vi "Variant to DBL.vi"(11 "Variant":variant) -> (2 "Value as DBL":dbl, 3 "Type":T1)   [LabVIEW 2022 SP3, in "Interlocks.lvlib"]
uses:
  Interlocks.lvlib
  Controls/Data Type.ctl
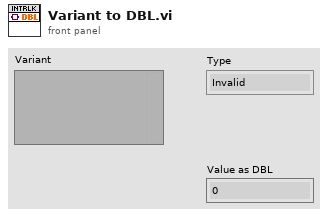
[diagram p1: front panel]
types:
  T1 = typedef "Interlocks.lvlib/Data Type.ctl" = enum8{"Invalid", "Boolean", "DBL", "I64", "U64"}
  T2 = enum8{"<Null>", "I8", "I16", "I32", "I64", "U8", "U16", "U32", "U64", "SGL", "DBL", "EXT", "CSG", "CDB", "CXT", "0x0F", "0x10", "0x11", "0x12", "0x13", "0x14", "Enum U8", "Enum U16", "Enum U32", "Enum U64", "SGL PQ", "DBL PQ", "EXT PQ", "CSG PQ", "CDB PQ", "CXT PQ", "0x1F", "0x20", "Boolean", "0x22", "0x23", "0x24", "0x25", "0x26", "0x27", "0x28", "0x29", "0x2A", "0x2B", "0x2C", "0x2D", "0x2E", "0x2F", "String", "0x31", "Path", "Pict", "0x34", "0x35", "0x36", "DAQ", "0x38", "0x39", "0x3A", "0x3B", "0x3C", "0x3D", "0x3E", "0x3F", "Array", "0x41", "0x42", "0x43", "0x44", "0x45", "0x46", "0x47", "0x48", "0x49", "0x4A", "0x4B", "0x4C", "0x4D", "0x4E", "0x4F", "Cluster", "0x51", "0x52", "Variant", "Waveform", "0x55", "0x56", "0x57", "0x58", "0x59", "0x5A", "0x5B", "0x5C", "0x5D", "0x5E", "Fixed Point", "0x60", "0x61", "0x62", "0x63", "0x64", "0x65", "0x66", "0x67", "0x68", "0x69", "0x6A", "0x6B", "0x6C", "0x6D", "0x6E", "0x6F", "Refnum", "0x71", "0x72", "Set Collection", "Map Collection"}
  T3 = cluster{"length":u16, "private":u8, "type":enum8{"<Null>", "I8", "I16", "I32", "I64", "U8", "U16", "U32", "U64", "SGL", "DBL", "EXT", "CSG", "CDB", "CXT", "0x0F", "0x10", "0x11", "0x12", "0x13", "0x14", "Enum U8", "Enum U16", "Enum U32", "Enum U64", "SGL PQ", "DBL PQ", "EXT PQ", "CSG PQ", "CDB PQ", "CXT PQ", "0x1F", "0x20", "Boolean", "0x22", "0x23", "0x24", "0x25", "0x26", "0x27", "0x28", "0x29", "0x2A", "0x2B", "0x2C", "0x2D", "0x2E", "0x2F", "String", "0x31", "Path", "Pict", "0x34", "0x35", "0x36", "DAQ", "0x38", "0x39", "0x3A", "0x3B", "0x3C", "0x3D", "0x3E", "0x3F", "Array", "0x41", "0x42", "0x43", "0x44", "0x45", "0x46", "0x47", "0x48", "0x49", "0x4A", "0x4B", "0x4C", "0x4D", "0x4E", "0x4F", "Cluster", "0x51", "0x52", "Variant", "Waveform", "0x55", "0x56", "0x57", "0x58", "0x59", "0x5A", "0x5B", "0x5C", "0x5D", "0x5E", "Fixed Point", "0x60", "0x61", "0x62", "0x63", "0x64", "0x65", "0x66", "0x67", "0x68", "0x69", "0x6A", "0x6B", "0x6C", "0x6D", "0x6E", "0x6F", "Refnum", "0x71", "0x72", "Set Collection", "Map Collection"}, "# elements":u16}
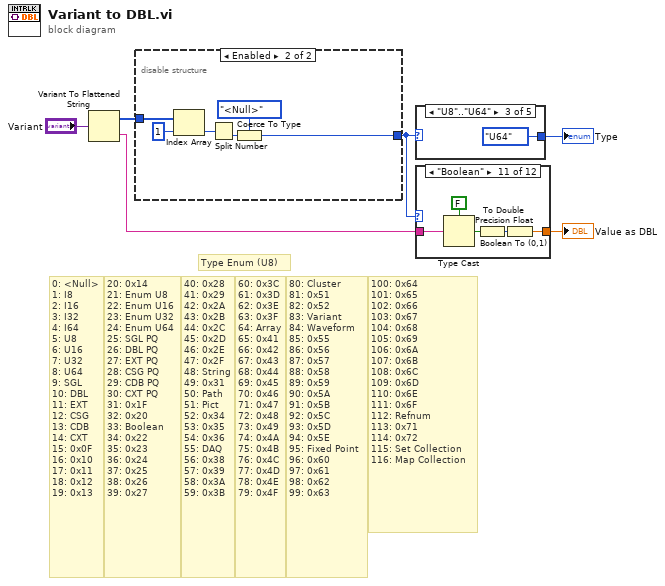
[diagram p0: block diagram]
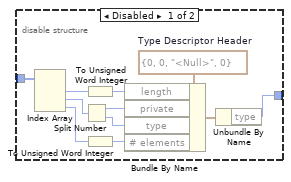
[diagram p2: hidden frame]
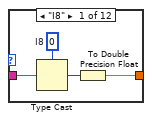
[diagram p3: hidden frame]
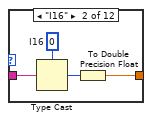
[diagram p4: hidden frame]
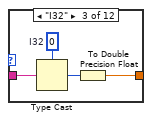
[diagram p5: hidden frame]
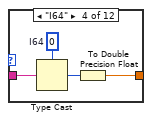
[diagram p6: hidden frame]
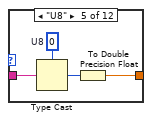
[diagram p7: hidden frame]
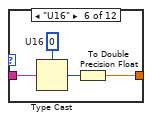
[diagram p8: hidden frame]
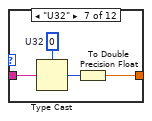
[diagram p9: hidden frame]
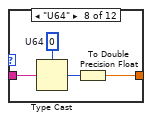
[diagram p10: hidden frame]
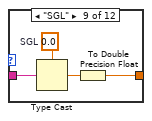
[diagram p11: hidden frame]
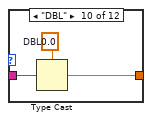
[diagram p12: hidden frame]
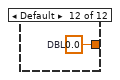
[diagram p13: hidden frame]
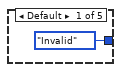
[diagram p14: hidden frame]
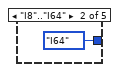
[diagram p15: hidden frame]
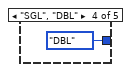
[diagram p16: hidden frame]
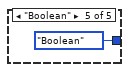
[diagram p17: hidden frame]
diagram:
  # "Type Enum (U8)"
  # "100: 0x64\n101: 0x65\n102: 0x66\n103: 0x67\n104: 0x68\n105: 0x69\n106: 0x6A\n107: 0x6B\n108: 0x6C\n109: 0x6D\n110: 0x6E\n111: 0x6F\n112: Refnum\n113: 0x71\n114: 0x72\n115: Set Collection\n116: Map Collection"
  # "80: Cluster\n81: 0x51\n82: 0x52\n83: Variant\n84: Waveform\n85: 0x55\n86: 0x56\n87: 0x57\n88: 0x58\n89: 0x59\n90: 0x5A\n91: 0x5B\n92: 0x5C\n93: 0x5D\n94: 0x5E\n95: Fixed Point\n96: 0x60\n97: 0x61\n98: 0x62\n99: 0x63"
  # "60: 0x3C\n61: 0x3D\n62: 0x3E\n63: 0x3F\n64: Array\n65: 0x41\n66: 0x42\n67: 0x43\n68: 0x44\n69: 0x45\n70: 0x46\n71: 0x47\n72: 0x48\n73: 0x49\n74: 0x4A\n75: 0x4B\n76: 0x4C\n77: 0x4D\n78: 0x4E\n79: 0x4F"
  # "40: 0x28\n41: 0x29\n42: 0x2A\n43: 0x2B\n44: 0x2C\n45: 0x2D\n46: 0x2E\n47: 0x2F\n48: String\n49: 0x31\n50: Path\n51: Pict\n52: 0x34\n53: 0x35\n54: 0x36\n55: DAQ\n56: 0x38\n57: 0x39\n58: 0x3A\n59: 0x3B"
  # "20: 0x14\n21: Enum U8\n22: Enum U16\n23: Enum U32\n24: Enum U64\n25: SGL PQ\n26: DBL PQ\n27: EXT PQ\n28: CSG PQ\n29: CDB PQ\n30: CXT PQ\n31: 0x1F\n32: 0x20\n33: Boolean\n34: 0x22\n35: 0x23\n36: 0x24\n37: 0x25\n38: 0x26 \n39: 0x27"
  # "0: <Null>\n1: I8\n2: I16\n3: I32\n4: I64\n5: U8\n6: U16\n7: U32\n8: U64\n9: SGL\n10: DBL\n11: EXT\n12: CSG\n13: CDB\n14: CXT\n15: 0x0F\n16: 0x10\n17: 0x11\n18: 0x12\n19: 0x13"
  n1 = Variant To Flattened String(Variant="Variant") -> (data string=w2:string, 1:w5:i16[])
  n2 = disable-structure shown="Enabled" {
    disable-tunnel: w5 -> [w9 w23]
    disable-tunnel: [w7 w18] -> w3
    frame Disabled {
      w12 = T3 {"length"=0, "private"=0, "type"=enum."<Null>", "# elements"=0}  # Type Descriptor Header
      n3 = Index Array(array=w9) -> (element #1=w13:i16, element #2=w16:i16, element #3=w17:i16)  [unwired: 3 in]
      n4 = Split Number(x=w16) -> (hi(x)=w14:u8, lo(x)=w15:u8)
      n5 = To Unsigned Word Integer(number=w13) -> (unsigned 16bit integer=w10:u16)
      n6 = To Unsigned Word Integer(number=w17) -> (unsigned 16bit integer=w11:u16)
      n7 = Bundle By Name(cluster=w12, "length"=w10, "private"=w14, "type"=w15, "# elements"=w11) -> (w8:T3)
      n8 = Unbundle By Name(w8) -> ("type"=w7:T2)
    }
    frame Enabled {
      n9 = Index Array(array=w23, index=1) -> (element=w21:i16)
      n10 = Split Number(x=w21) -> (lo(x)=w20:u8)  [unwired: 1 out]
      n11 = Coerce To Type(0:w20, 1:T2."<Null>" ("type")) -> (2:w18:T2)
    }
  }
  n12 = case shown="\"U8\"..\"U64\"" w3 {
    tunnel: [Data_Type."Invalid" ("Type") Data_Type."I64" ("Type") Data_Type."U64" ("Type") Data_Type."DBL" ("Type") Data_Type."Boolean" ("Type")] -> w4
    frame Default {
    }
    frame "I8".."I64" {
    }
    frame "U8".."U64" {
    }
    frame "SGL", "DBL" {
    }
    frame "Boolean" {
    }
  }
  "Type" <- w4
  n13 = case shown="\"Boolean\"" w3 {
    tunnel: w2 -> [w32 w36 w40 w43 w48 w52 w56 w60 w64 w66 w72 _]
    tunnel: [w29 w33 w37 w41 w45 w49 w53 w57 w61 w65 w68 w73] -> w1
    frame "I8" {
      w31 = i8 0  # I8
      n14 = Type Cast(type=w31, x=w32) -> (*(type *) &x=w30:i8)
      n15 = To Double Precision Float(number=w30) -> (double precision float=w29:dbl)
    }
    frame "I16" {
      w35 = i16 0  # I16
      n16 = Type Cast(type=w35, x=w36) -> (*(type *) &x=w34:i16)
      n17 = To Double Precision Float(number=w34) -> (double precision float=w33:dbl)
    }
    frame "I32" {
      w39 = 0  # I32
      n18 = Type Cast(type=w39, x=w40) -> (*(type *) &x=w38:i32)
      n19 = To Double Precision Float(number=w38) -> (double precision float=w37:dbl)
    }
    frame "I64" {
      w44 = i64 0  # I64
      n20 = Type Cast(type=w44, x=w43) -> (*(type *) &x=w42:i64)
      n21 = To Double Precision Float(number=w42) -> (double precision float=w41:dbl)
    }
    frame "U8" {
      w47 = u8 0  # U8
      n22 = Type Cast(type=w47, x=w48) -> (*(type *) &x=w46:u8)
      n23 = To Double Precision Float(number=w46) -> (double precision float=w45:dbl)
    }
    frame "U16" {
      w51 = u16 0  # U16
      n24 = Type Cast(type=w51, x=w52) -> (*(type *) &x=w50:u16)
      n25 = To Double Precision Float(number=w50) -> (double precision float=w49:dbl)
    }
    frame "U32" {
      w55 = u32 0  # U32
      n26 = Type Cast(type=w55, x=w56) -> (*(type *) &x=w54:u32)
      n27 = To Double Precision Float(number=w54) -> (double precision float=w53:dbl)
    }
    frame "U64" {
      w59 = u64 0  # U64
      n28 = Type Cast(type=w59, x=w60) -> (*(type *) &x=w58:u64)
      n29 = To Double Precision Float(number=w58) -> (double precision float=w57:dbl)
    }
    frame "SGL" {
      w63 = sgl 0.0  # SGL
      n30 = Type Cast(type=w63, x=w64) -> (*(type *) &x=w62:sgl)
      n31 = To Double Precision Float(number=w62) -> (double precision float=w61:dbl)
    }
    frame "DBL" {
      w67 = 0.0  # DBL
      n32 = Type Cast(type=w67, x=w66) -> (*(type *) &x=w65:dbl)
    }
    frame "Boolean" {
      n33 = Type Cast(type=FALSE, x=w72) -> (*(type *) &x=w70:bool)
      n34 = Boolean To (0,1)(Boolean=w70) -> (0, 1=w69:i16)
      n35 = To Double Precision Float(number=w69) -> (double precision float=w68:dbl)
    }
    frame Default {
      w73 = 0.0  # DBL
    }
  }
  "Value as DBL" <- w1
